vi "CALC_CORR_EDEL_TIME.vi"(0 "VISA IN":refnum<visa-resource-name>, 1 "Delay(sec)":dbl, 5 "error in":errorcluster, 7 "Channel":i32) -> (14 "VISA Out":refnum<visa-resource-name>, 19 "error out":errorcluster)   [LabVIEW 2018, in "PNA-X.lvlib"]
doc: "CALCulate<cnum>:CORRection:EDELay:TIME <num> \n(Read-Write) Sets the electrical delay for the selected measurement. \nSee Critical Note \nParameters \n<cnum> Channel number of the measurement. There must be a selected measurement \non that channel. If unspecified, <cnum> is set to 1. \n<num> Electrical delay in seconds. Choose any number between: \n-10.00 and 10.00 \nUse SENS:CORR:RVEL:COAX <num> to set Velocity factor. \nExamples CALC1:CORR:EDEL:TIME 1NS \ncalculate2:correction:time 0.5e-12 \nQuery Syntax CALCulate:CORRection:EDELay:TIME? \nReturn Type Numeric \nDefault 0 seconds"
uses:
  PNA-X.lvlib
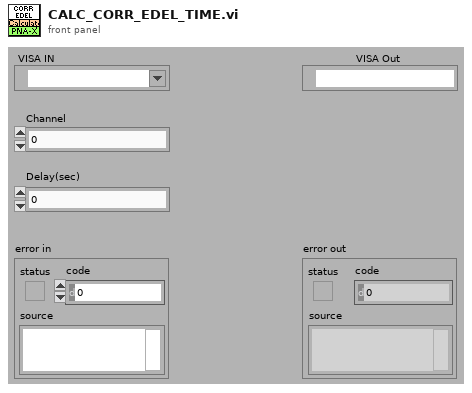
[diagram p1: front panel]
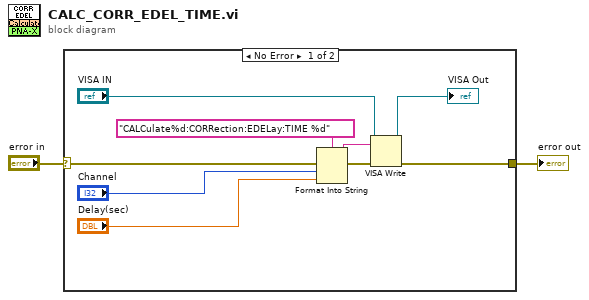
[diagram p0: block diagram]
diagram:
  n1 = case shown="No Error" "error in" {
    selector: "error in" -> [w11 w12]
    tunnel: [w6 w12] -> w1
    frame No Error {
      n2 = Format Into String(format string="CALCulate%d:CORRection:EDELay:TIME %d" ("Cmdline"), error in=w11, "Channel", "Delay(sec)") -> (resulting string=w9:string, error out=w10:errorcluster)  [unwired: 1 in]
      n3 = VISA Write(VISA resource name="VISA IN", write buffer=w9, error in (no error)=w10) -> (VISA resource name out=→"VISA Out":refnum<visa-resource-name>, error out=w6:errorcluster)  [unwired: 1 out]
    }
    frame Error {
    }
  }
  "error out" <- w1
